vi "Scale Value.vi"(10 "Limits":T1, 11 "Value":dbl format="%#_13g") -> (3 "Scaled Value":dbl)   [LabVIEW 2019, in "Audio Processing.lvlib"]
doc: "Scale the input value to the range defined by Limits. Assumes the input value is in range 0-127. Any scaled values outside the limit range will be clamped to the upper or lower limit."
uses:
  Audio Processing.lvlib
  Value Properties.ctl
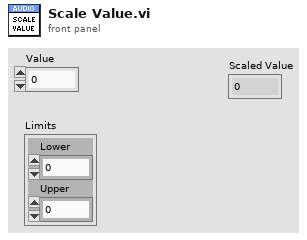
[diagram p1: front panel]
types:
  T1 = typedef "Audio Processing.lvlib/Value Properties.ctl" = cluster{"Lower":dbl, "Upper":dbl}
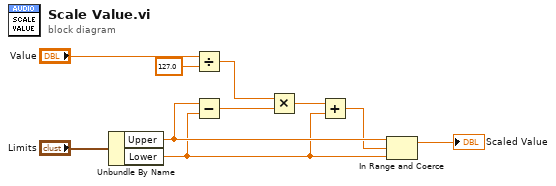
[diagram p0: block diagram]
diagram:
  n1 = Unbundle By Name("Limits") -> ("Upper"=w4:dbl, "Lower"=w2:dbl)
  n2 = Divide(x="Value", y=127.0) -> (x/y=w5:dbl)
  n3 = Subtract(x=w4, y=w2) -> (x-y=w9:dbl)
  n4 = Multiply(x=w5, y=w9) -> (x*y=w8:dbl)
  n5 = Add(x=w8, y=w2) -> (x+y=w3:dbl)
  n6 = In Range and Coerce(upper limit=w4, x=w3, lower limit=w2) -> (coerced(x)=→"Scaled Value":dbl)  [unwired: 1 out]
